vi "Microscope.CreateDependencies.vi"(8 "error in (no error)":errorcluster, 11 "Microscope in":refnum<class "Microscope.lvclass">) -> (0 "error out":errorcluster, 3 "Microscope out":refnum<class "Microscope.lvclass">)   [LabVIEW 2015, in "Microscope.lvclass"]
uses:
  Microscope.lvclass
  <vilib>/JKI/JKI SMO/SMO/SMO.lvclass
  XYStage/XYStage.lvclass
  Camera/Camera.lvclass
  Camera.Simulated/Camera.Simulated.lvclass
  Camera.IMAQdx/Camera.IMAQdx.lvclass
  XYStage.Simulated/XYStage.Simulated.lvclass
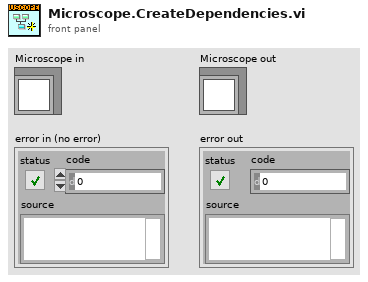
[diagram p1: front panel]
types:
  T1 = typedef "Microscope.lvclass/Configuration--Cluster.ctl" = cluster{"XY Stage":string, "Camera":string, "image output folder":path, "filetype":string}
  T2 = typedef "Microscope.lvclass/Dependencies--Cluster.ctl" = cluster{"XYStage":refnum<class "XYStage.lvclass">, "Camera":refnum<class "Camera.lvclass">}
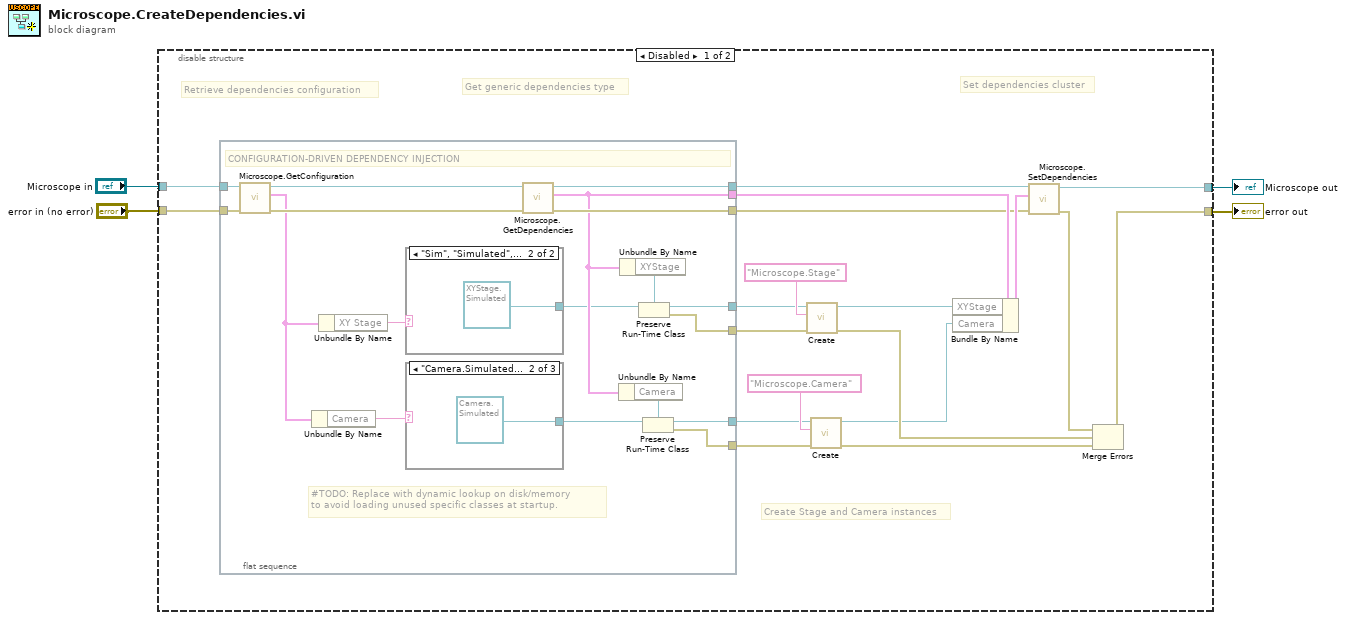
[diagram p0: block diagram]
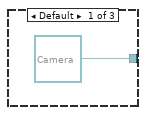
[diagram p2: hidden frame]
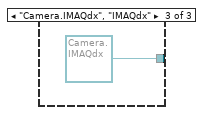
[diagram p3: hidden frame]
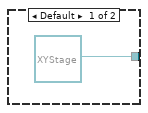
[diagram p4: hidden frame]
diagram:
  n1 = disable-structure shown="Disabled" {
    disable-tunnel: [w23 w47] -> w4
    disable-tunnel: "error in (no error)" -> [w21 w47]
    disable-tunnel: "Microscope in" -> [w20 w48]
    disable-tunnel: [w6 w48] -> w1
    frame Disabled {
      # "Set dependencies cluster"
      # "Create Stage and Camera instances"
      # "Get generic dependencies type"
      # "Retrieve dependencies configuration"
      n2 = flat-sequence {
        tunnel: w20 -> [w41]
        tunnel: w21 -> [w40]
        tunnel: [w39] -> w5
        tunnel: [w37] -> w7
        tunnel: [w35] -> w9
        tunnel: [w30] -> w12
        tunnel: [w27] -> w13
        tunnel: [w25] -> w14
        tunnel: [w24] -> w15
        frame #0 {
          # "#TODO: Replace with dynamic lookup on disk/memory\nto avoid loading unused specific classes at startup."
          # "CONFIGURATION-DRIVEN DEPENDENCY INJECTION"
          n3 = call "Microscope.GetConfiguration.vi"("error in (no error)"=w40, "Microscope"=w41) -> ("error out"=w36:errorcluster, "Configuration"=w34:T1, "Microscope out"=w38:refnum<class "Microscope.lvclass">)  [unwired: 7 in]
          n4 = Unbundle By Name(w34) -> ("Camera"=w32:string)
          n5 = Unbundle By Name(w34) -> ("XY Stage"=w33:string)
          n6 = case shown="\"Sim\", \"Simulated\", \"XYStage.Simulated\"" w33 {
            tunnel: [refnum<class "XYStage.lvclass"> refnum ("XYStage.lvclass") refnum<class "XYStage.Simulated.lvclass"> refnum ("XYStage.Simulated.lvclass")] -> w29
            frame Default {
            }
            frame "Sim", "Simulated", "XYStage.Simulated" {
            }
          }
          n7 = case shown="\"Camera.Simulated\", \"Sim\", \"Simulated\"" w32 {
            tunnel: [refnum<class "Camera.lvclass"> refnum ("Camera.lvclass") refnum<class "Camera.Simulated.lvclass"> refnum ("Camera.Simulated.lvclass") refnum<class "Camera.IMAQdx.lvclass"> refnum ("Camera.IMAQdx.lvclass")] -> w26
            frame Default {
            }
            frame "Camera.Simulated", "Sim", "Simulated" {
            }
            frame "Camera.IMAQdx", "IMAQdx" {
            }
          }
          n8 = call "Microscope.GetDependencies.vi"("error in (no error)"=w36, "Microscope"=w38) -> ("error out"=w37:errorcluster, "Dependencies"=w35:T2, "Microscope out"=w39:refnum<class "Microscope.lvclass">)  [unwired: 7 in]
          n9 = Unbundle By Name(w35) -> ("Camera"=w28:refnum<class "Camera.lvclass">)
          n10 = Unbundle By Name(w35) -> ("XYStage"=w31:refnum<class "XYStage.lvclass">)
          n11 = Preserve Run-Time Class(object in=w29, 2:w31) -> (object out=w30:refnum<class "XYStage.lvclass">, error out=w25:errorcluster)  [unwired: 1 in]
          n12 = Preserve Run-Time Class(object in=w26, 2:w28) -> (object out=w27:refnum<class "Camera.lvclass">, error out=w24:errorcluster)  [unwired: 1 in]
        }
      }
      n13 = call <vilib>:"Create.vi"("error in (no error)"=w14, "Subsystem Name (optional)"="Microscope.Stage", "SMO"=w12) -> ("error out"=w19:errorcluster, "SMO out"=w10:refnum<class "XYStage.lvclass">)  [unwired: 6 in, 1 out]
      n14 = call <vilib>:"Create.vi"("error in (no error)"=w15, "Subsystem Name (optional)"="Microscope.Camera", "SMO"=w13) -> ("error out"=w18:errorcluster, "SMO out"=w11:refnum<class "Camera.lvclass">)  [unwired: 6 in, 1 out]
      n15 = Bundle By Name(cluster=w9, "XYStage"=w10, "Camera"=w11) -> (w8:T2)
      n16 = call "Microscope.SetDependencies.vi"("error in (no error)"=w7, "Dependencies"=w8, "Microscope"=w5) -> ("error out"=w22:errorcluster, "Microscope out"=w6:refnum<class "Microscope.lvclass">)  [unwired: 7 in]
      n17 = Merge Errors(w22, w19, w18) -> (w23:errorcluster)
    }
    frame Enabled {
    }
  }
  "error out" <- w4
  "Microscope out" <- w1
